vi "FN.vi"(0 "Offset_h":fxp<+/-,32,8>, 1 "Offset_out":fxp<+/-,32,8>, 2 "Inputs":fxp<+/-,32,8>[](array[numeric]), 3 "Weights_h":fxp<+/-,32,8>[][](array[numeric]), 4 "Weights_out":fxp<+/-,32,8>[][](array[numeric])) -> (5 "Outputs_hx":fxp<+/-,32,8>[](array[numeric]), 6 "Outputs_out":fxp<+/-,32,8>[](array[numeric]))   [LabVIEW 2016]
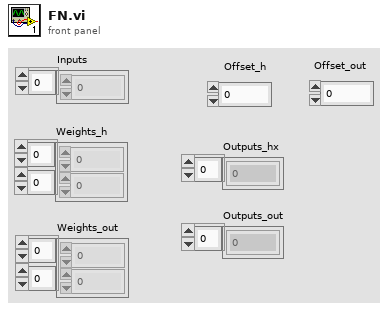
[diagram p1: front panel]
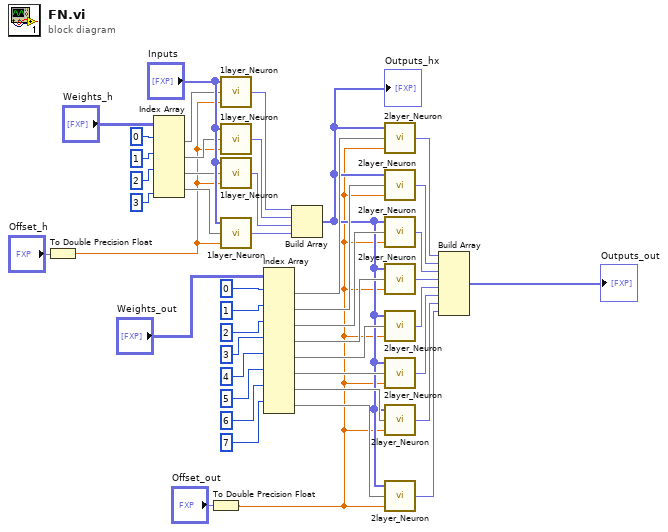
[diagram p0: block diagram]
diagram:
  n1 = To Double Precision Float(number="Offset_h") -> (double precision float=w3:dbl)
  n2 = Index Array(array="Weights_h", index (row) #1=0 ("index (row)"), index (row) #2=1 ("index (row)"), index (row) #3=2 ("index (row)"), index (col) #4=3 ("disabled index (col)")) -> (element #1=w35:fxp<+/-,32,8>[], element #2=w34:fxp<+/-,32,8>[], element #3=w33:fxp<+/-,32,8>[], element #4=w32:fxp<+/-,32,8>[])  [unwired: 4 in]
  n3 = To Double Precision Float(number="Offset_out") -> (double precision float=w1:dbl)
  n4 = call "1layer_Neuron.vi"("Offset"=w3, "Weights"=w35, "Inputs"="Inputs") -> ("Output"=w44:fxp<+/-,32,8>)
  n5 = call "1layer_Neuron.vi"("Offset"=w3, "Weights"=w34, "Inputs"="Inputs") -> ("Output"=w43:fxp<+/-,32,8>)
  n6 = call "1layer_Neuron.vi"("Offset"=w3, "Weights"=w33, "Inputs"="Inputs") -> ("Output"=w42:fxp<+/-,32,8>)
  n7 = call "1layer_Neuron.vi"("Offset"=w3, "Weights"=w32, "Inputs"="Inputs") -> ("Output"=w41:fxp<+/-,32,8>)
  n8 = Index Array(array="Weights_out", index (row) #1=0 ("index (row)"), index (row) #2=1 ("index (row)"), index (row) #3=2 ("index (row)"), index (row) #4=3 ("disabled index (col)"), index (row) #5=4 ("index (row)"), index (row) #6=5 ("index (row)"), index (row) #7=6 ("index (row)"), index (row) #8=7 ("disabled index (col)")) -> (element #1=w22:fxp<+/-,32,8>[], element #2=w21:fxp<+/-,32,8>[], element #3=w20:fxp<+/-,32,8>[], element #4=w19:fxp<+/-,32,8>[], element #5=w18:fxp<+/-,32,8>[], element #6=w17:fxp<+/-,32,8>[], element #7=w16:fxp<+/-,32,8>[], element #8=w15:fxp<+/-,32,8>[])  [unwired: 8 in]
  n9 = Build Array(w44, w43, w42, w41) -> (w5:fxp<+/-,32,8>[])
  "Outputs_hx" <- w5
  n10 = call "2layer_Neuron.vi"("Offset"=w1, "Weights_2layer"=w22, "Array_Out_hx"=w5) -> ("Output"=w13:fxp<+/-,32,8>)
  n11 = call "2layer_Neuron.vi"("Offset"=w1, "Weights_2layer"=w21, "Array_Out_hx"=w5) -> ("Output"=w12:fxp<+/-,32,8>)
  n12 = call "2layer_Neuron.vi"("Offset"=w1, "Weights_2layer"=w20, "Array_Out_hx"=w5) -> ("Output"=w11:fxp<+/-,32,8>)
  n13 = call "2layer_Neuron.vi"("Offset"=w1, "Weights_2layer"=w19, "Array_Out_hx"=w5) -> ("Output"=w10:fxp<+/-,32,8>)
  n14 = call "2layer_Neuron.vi"("Offset"=w1, "Weights_2layer"=w18, "Array_Out_hx"=w5) -> ("Output"=w9:fxp<+/-,32,8>)
  n15 = call "2layer_Neuron.vi"("Offset"=w1, "Weights_2layer"=w17, "Array_Out_hx"=w5) -> ("Output"=w8:fxp<+/-,32,8>)
  n16 = call "2layer_Neuron.vi"("Offset"=w1, "Weights_2layer"=w16, "Array_Out_hx"=w5) -> ("Output"=w7:fxp<+/-,32,8>)
  n17 = call "2layer_Neuron.vi"("Offset"=w1, "Weights_2layer"=w15, "Array_Out_hx"=w5) -> ("Output"=w6:fxp<+/-,32,8>)
  n18 = Build Array(w13, w12, w11, w10, w9, w8, w7, w6) -> (→"Outputs_out":fxp<+/-,32,8>[])
